vi "Volt Range.vi"() -> ()   [LabVIEW 2020, in "Yokogawa GX Series.lvlib"]
uses:
  <instrlib>/Yokogawa GX Series/Yokogawa GX Series.lvlib
panel:
  in  "Volt Range":string="20mV\n60mV\n200mV\n1V\n2V\n6V\n20V\n50V"
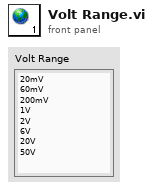
[diagram p1: front panel]
diagram:
